vi "Notifer-base.vi"() -> ()   [LabVIEW 2020]
doc: "Use this template to build a master/slave design pattern. The master loop always executes. It notifies one or more slave loops to execute their code. The slave loop(s) continue executing until they complete, then wait for another notification. Contrast this with the Producer/Consumer pattern in which the consumer loops execute only when they have data in their queue."
panel:
  in  "Start":bool
  in  "stop":bool
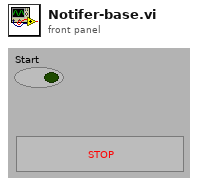
[diagram p1: front panel]
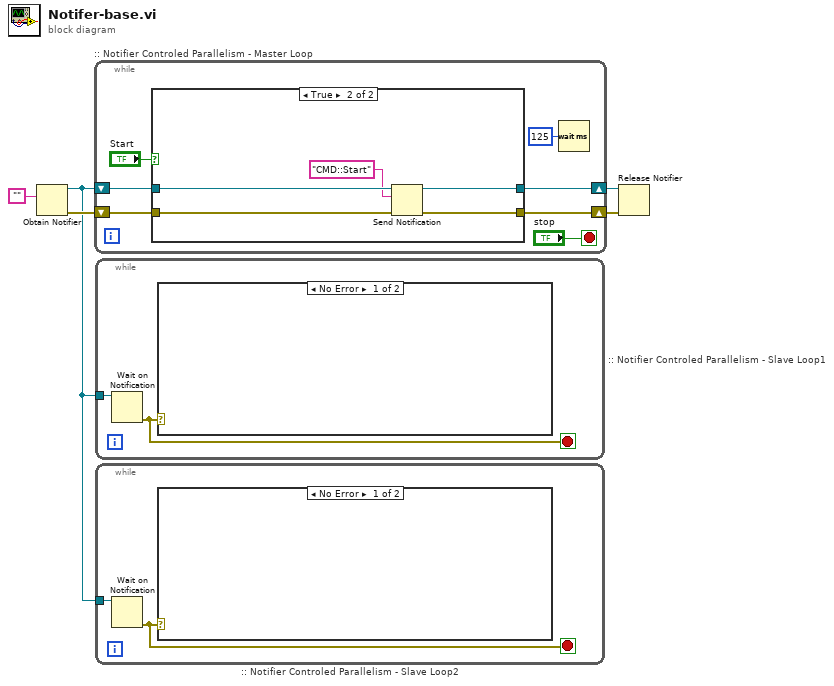
[diagram p0: block diagram]
diagram:
  n1 = Obtain Notifier(notification data type="" ("data (can be any type)")) -> (notifier out=w1:refnum<notifier>, error out=w5:errorcluster)  [unwired: 2 in, 2 out]
  n2 = while ":: Notifier Controled Parallelism - Master Loop" {
    shift-right: [w10] -> w4
    shift-left: w5 -> [w9]
    shift-right: [w8] -> w3
    shift-left: w1 -> [w11]
    stop <- "stop" stop-if-true
    n3 = case shown="True" "Start" {
      tunnel: w11 -> [w14 w19]
      tunnel: [w13 w18] -> w10
      tunnel: w9 -> [w13 w17]
      tunnel: [w14 w16] -> w8
      frame False {
      }
      frame True {
        n4 = Send Notification(notification="CMD::Start", notifier=w19, error in (no error)=w17) -> (notifier out=w16:refnum<notifier>, error out=w18:errorcluster)
      }
    }
    n5 = Wait (ms)(milliseconds to wait=u32 125) -> ()  [unwired: 1 out]
  }
  n6 = while ":: Notifier Controled Parallelism - Slave Loop1" {
    tunnel: w1 -> [w21]
    stop <- w20 stop-if-true
    n7 = Wait on Notification(notifier=w21) -> (error out=w20:errorcluster)  [unwired: 1 in, 5 out]
    n8 = case shown="No Error" w20 {
      frame No Error {
      }
      frame Error {
      }
    }
  }
  n9 = while ":: Notifier Controled Parallelism - Slave Loop2" {
    tunnel: w1 -> [w23]
    stop <- w22 stop-if-true
    n10 = Wait on Notification(notifier=w23) -> (error out=w22:errorcluster)  [unwired: 1 in, 5 out]
    n11 = case shown="No Error" w22 {
      frame No Error {
      }
      frame Error {
      }
    }
  }
  n12 = Release Notifier(notifier=w3, error in (no error)=w4) -> ()  [unwired: 4 out]
